vi "IsSessionLoaded.vi"(7 "DLL path":path, 8 "error in (no error)":errorcluster, 11 "session id in":i32) -> (0 "error out":errorcluster, 2 "Is Loaded":bool, 3 "session id out":i32)   [LabVIEW 2017, in "ONNX Class Library.lvlib"]
doc: "/**\n * @brief Проверить, загружена ли сессия в память\n * \n * Функция возвращает текущий статус сессии. Полезно для проверки перед вызовом\n * инференса, особенно если использовалась функция UnloadSession.\n * \n * @param sessionId [IN] ID сессии, полученный от CreateSession\n * \n * @return int32: 1 если сессия активна и модель загружена в память\n * @return int32: 0 если сессия не найдена или выгружена из памяти\n */\nint IsSessionLoaded(int sessionId);"
uses:
  ONNX Class Library.lvlib
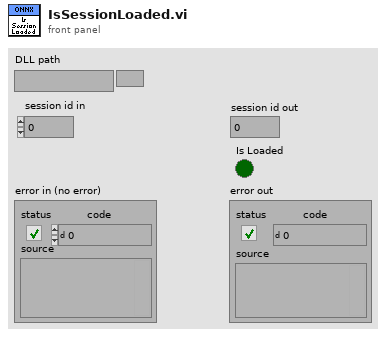
[diagram p1: front panel]
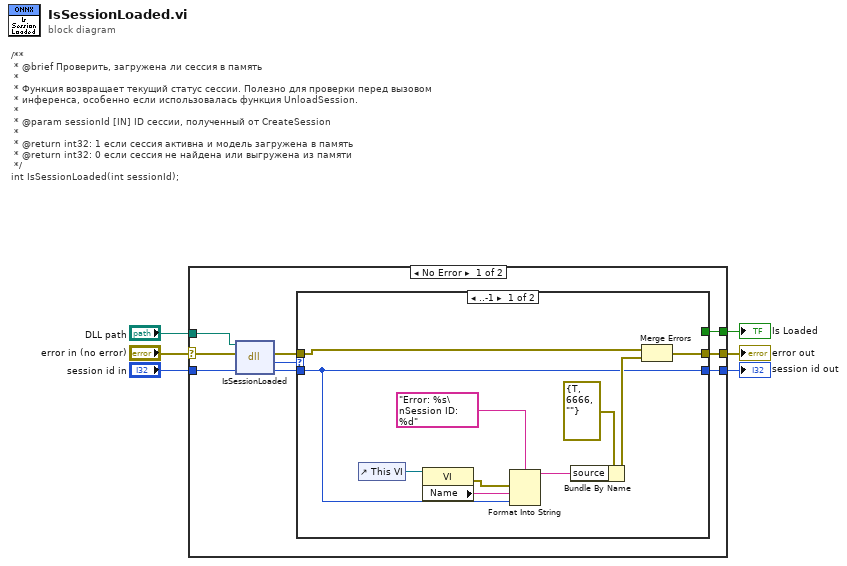
[diagram p0: block diagram]
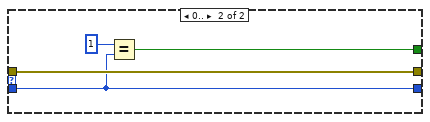
[diagram p2: hidden frame]
diagram:
  # "/**\n * @brief Проверить, загружена ли сессия в память\n * \n * Функция возвращает текущий статус сессии. Полезно для проверки перед вызовом\n * инференса, особенно если использовалась функция UnloadSession.\n * \n * @param sessionId [IN] ID сессии, полученный от CreateSession\n * \n * @return int32: 1 если сессия активна и модель загружена в память\n * @return int32: 0 если сессия не найдена или выгружена из памяти\n */\nint IsSessionLoaded(int sessionId);"
  n1 = case shown="No Error" "error in (no error)" {
    selector: "error in (no error)" -> [w8 w31]
    tunnel: "session id in" -> [w15 w30]
    tunnel: [w11 w31] -> w5
    tunnel: [w10 w30] -> w4
    tunnel: [w9 _] -> w3
    tunnel: "DLL path" -> [w7 _]
    frame No Error {
      n2 = dll-call lib="home/ivan/LabVIEWData/ONNX/Test/libonnx_wrapper/unix64/libonnx_wrapper.so" fn="IsSessionLoaded"(path in=w7, error in=w8, "sessionId"=w15) -> (error out=w14:errorcluster, "return"=w13:i32, "sessionId"=w12:i32)  [unwired: 1 in, 1 out]
      n3 = case shown="..-1" w13 {
        tunnel: w14 -> [w16 w29]
        tunnel: [w17 w29] -> w11
        tunnel: w12 -> [w18 w28]
        tunnel: [w18 w28] -> w10
        tunnel: [_ w26] -> w9
        frame ..-1 {
          n4 = control-ref of="This VI"() -> (w22:refnum<vi>)
          n5 = property class="VI"(reference=w22) -> (error out=w19:errorcluster, "Name"=w21:string)  [unwired: 1 in, 1 out]
          n6 = Format Into String(format string="Error: %s\nSession ID: %d", error in=w19, w21, w18) -> (resulting string=w23:string)  [unwired: 1 in, 1 out]
          n7 = Bundle By Name(cluster=errorcluster {"status"=TRUE, "code"=6666, "source"=""} ("error out"), "source"=w23) -> (w24:errorcluster)
          n8 = Merge Errors(w16, w24) -> (w17:errorcluster)
        }
        frame 0.. {
          n9 = Equal?(x=1, y=w28) -> (x = y?=w26:bool)
        }
      }
    }
    frame Error {
    }
  }
  "error out" <- w5
  "session id out" <- w4
  "Is Loaded" <- w3
